vi "updateGraphs.vi"(8 "error in (no error)":errorcluster, 10 "Array":dbl[](array[numeric]), 11 "AnalysisResultsViewer in":refnum<class "AnalysisResultsViewer.lvclass">) -> (0 "error out":errorcluster, 3 "AnalysisResultsViewer out":refnum<class "AnalysisResultsViewer.lvclass">)   [LabVIEW 2009, in "Views.lvlib" / "Camera.lvlib" / "AnalysisResultsViewer.lvclass"]
uses:
  AnalysisResultsViewer.lvclass
  AnalysisResultsViewer.lvclass/AnalysisResultsViewer.ctl
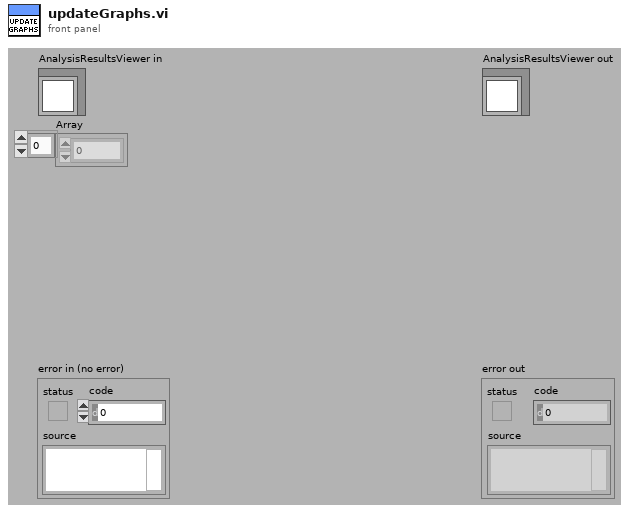
[diagram p1: front panel]
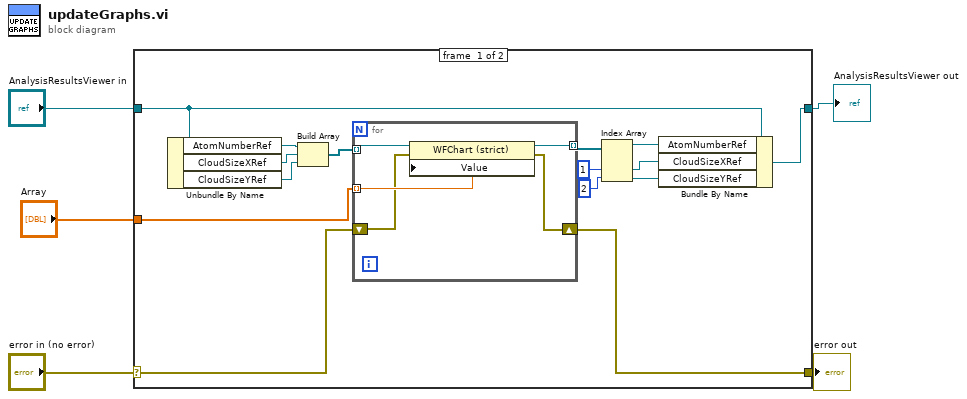
[diagram p0: block diagram]
diagram:
  n1 = case shown="No Error" "error in (no error)" {
    selector: "error in (no error)" -> [w9 w27]
    tunnel: [w8 w27] -> w4
    tunnel: [w6 w26] -> w2
    tunnel: "AnalysisResultsViewer in" -> [w7 w26]
    tunnel: "Array" -> [w10 _]
    frame #0 {
      n2 = Unbundle By Name(w7) -> ("AtomNumberRef"=w13:refnum<vi>, "CloudSizeXRef"=w12:refnum<vi>, "CloudSizeYRef"=w11:refnum<vi>)
      n3 = Build Array(w13, w12, w11) -> (w20:refnum<vi>[])
      n4 = for {
        tunnel: w20 -> [w25] mode=indexing
        tunnel: w10 -> [w24] mode=indexing
        tunnel: [w21] -> w19 mode=indexing
        shift-right: [w22] -> w8
        shift-left: w9 -> [w23]
        n5 = property class="WFChart (strict)"(reference=w25, error in=w23, "Value"=w24) -> (reference out=w21:refnum<vi>, error out=w22:errorcluster)
      }
      n6 = Index Array(array=w19, index #2=1, index #3=2) -> (element #1=w18:refnum<vi>, element #2=w16:refnum<vi>, element #3=w17:refnum<vi>)  [unwired: 1 in]
      n7 = Bundle By Name(cluster=w7, "AtomNumberRef"=w18, "CloudSizeXRef"=w16, "CloudSizeYRef"=w17) -> (w6:refnum<class "AnalysisResultsViewer.lvclass">)
    }
    frame #1 {
    }
  }
  "error out" <- w4
  "AnalysisResultsViewer out" <- w2
